vi "RichToFlatcif_manager_PluginInfoArray.vi"(5 "OutputClusterType":T1, 11 "InputCluster":T15) -> (3 "OutputCluster":T1)   [LabVIEW 2021, in "CIF_Manager_server.lvlib"]
uses:
  CIF_Manager_server.lvlib
  cif_manager_PluginInfoArray.ctl
  cif_manager_PluginInfo.ctl
  cif_common_ShortVersion.ctl
  cif_management_common_PluginStatusData.ctl
  cif_management_common_PluginStatusData_PluginState.ctl
  cif_management_common_TimingStatistics.ctl
  cif_common_TimingStats.ctl
  cif_management_common_FifoStatistics.ctl
  cif_management_common_Error.ctl
  cif_management_common_MonitorDoubles.ctl
  cif_management_common_MonitorU64.ctl
  cif_management_common_MonitorI64.ctl
  cif_management_common_LoaderInfo.ctl
  cif_management_common_LoaderType.ctl
  cif_manager_PluginInfoArray_Flat.ctl
  cif_manager_PluginInfo_Flat.ctl
  cif_common_ShortVersion_Flat.ctl
  cif_management_common_PluginStatusData_Flat.ctl
  cif_management_common_TimingStatistics_Flat.ctl
  cif_common_TimingStats_Flat.ctl
  cif_management_common_FifoStatistics_Flat.ctl
  cif_management_common_Error_Flat.ctl
  cif_management_common_MonitorDoubles_Flat.ctl
  cif_management_common_MonitorU64_Flat.ctl
  cif_management_common_MonitorI64_Flat.ctl
  cif_management_common_LoaderInfo_Flat.ctl
  RichToFlatcif_common_ShortVersion.vi
  RichToFlatcif_management_common_PluginStatusData.vi
  RichToFlatcif_management_common_LoaderInfo.vi
  RichToFlatcif_management_common_TimingStatistics.vi
  RichToFlatcif_management_common_FifoStatistics.vi
  RichToFlatcif_management_common_Error.vi
  RichToFlatcif_management_common_MonitorDoubles.vi
  RichToFlatcif_management_common_MonitorU64.vi
  RichToFlatcif_management_common_MonitorI64.vi
  RichToFlatcif_common_TimingStats.vi
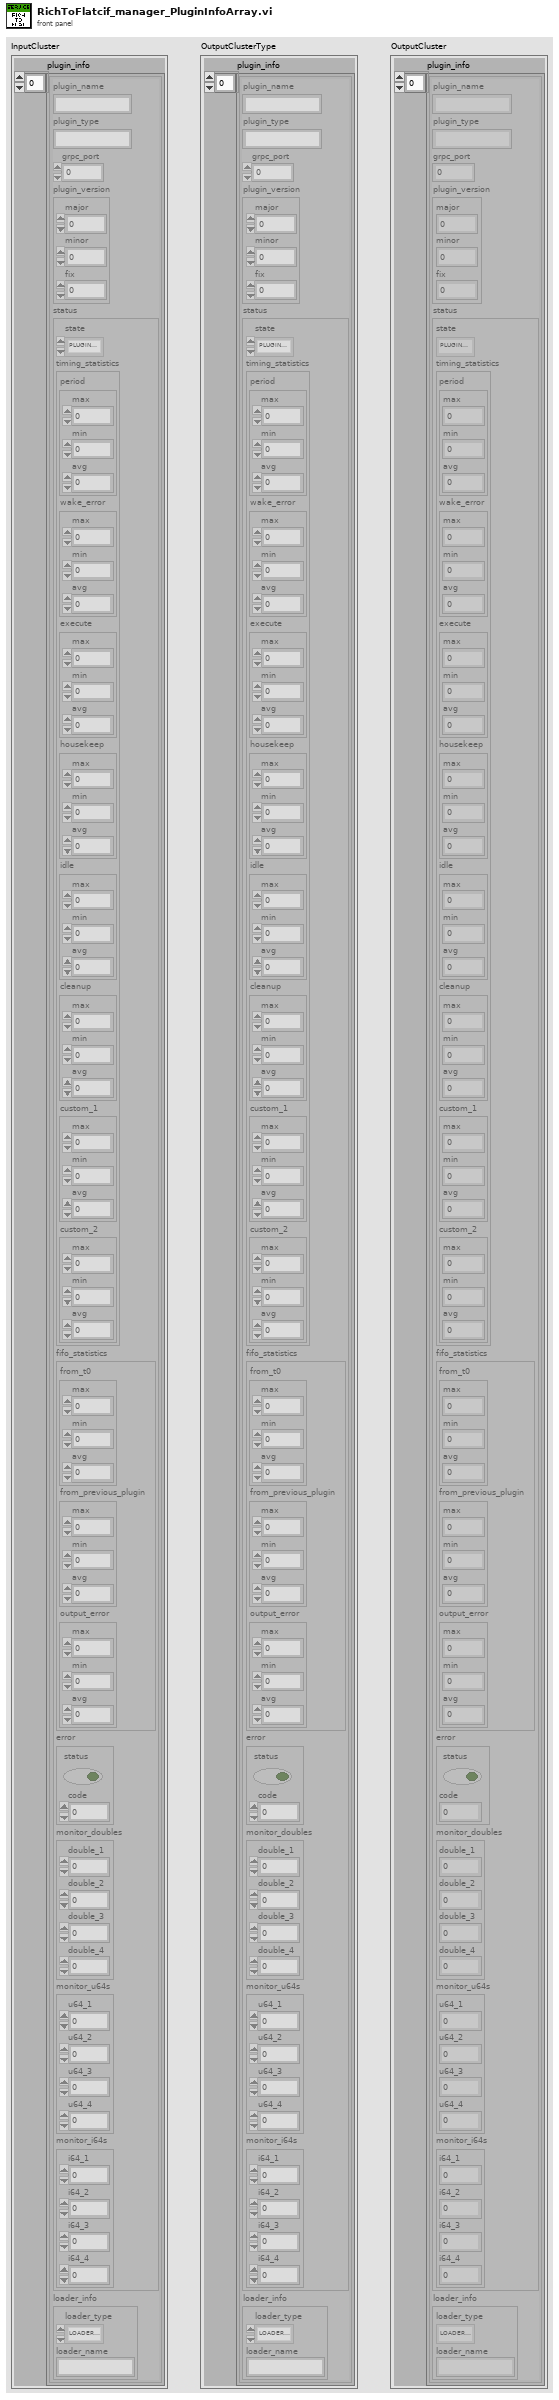
[diagram p1: front panel]
types:
  T1 = typedef "CIF_Manager_server.lvlib/cif_manager_PluginInfoArray_Flat.ctl" = cluster{"plugin_info":T2[]}
  T2 = typedef "CIF_Manager_server.lvlib/cif_manager_PluginInfo_Flat.ctl" = cluster{"plugin_name":string, "plugin_type":string, "grpc_port":i32, "plugin_version":T3, "status":T4, "loader_info":T13}
  T3 = typedef "CIF_Manager_server.lvlib/cif_common_ShortVersion_Flat.ctl" = cluster{"major":u32, "minor":u32, "fix":u32}
  T4 = typedef "CIF_Manager_server.lvlib/cif_management_common_PluginStatusData_Flat.ctl" = cluster{"state":T5, "timing_statistics":T6, "fifo_statistics":T8, "error":T9, "monitor_doubles":T10, "monitor_u64s":T11, "monitor_i64s":T12}
  T5 = typedef "CIF_Manager_server.lvlib/cif_management_common_PluginStatusData_PluginState.ctl" = enum32{"PLUGINSTATE_UNKNOWN", "PLUGINSTATE_CREATING", "PLUGINSTATE_LISTENING", "PLUGINSTATE_RUNNING", "PLUGINSTATE_CLEANINGUP", "PLUGINSTATE_DESTROYING", "PLUGINSTATE_PREPARED", "PLUGINSTATE_FTE_RUN"}
  T6 = typedef "CIF_Manager_server.lvlib/cif_management_common_TimingStatistics_Flat.ctl" = cluster{"period":T7, "wake_error":T7, "execute":T7, "housekeep":T7, "idle":T7, "cleanup":T7, "custom_1":T7, "custom_2":T7}
  T7 = typedef "CIF_Manager_server.lvlib/cif_common_TimingStats_Flat.ctl" = cluster{"max":i64, "min":i64, "avg":dbl}
  T8 = typedef "CIF_Manager_server.lvlib/cif_management_common_FifoStatistics_Flat.ctl" = cluster{"from_t0":T7, "from_previous_plugin":T7, "output_error":T7}
  T9 = typedef "CIF_Manager_server.lvlib/cif_management_common_Error_Flat.ctl" = cluster{"status":bool, "code":i32}
  T10 = typedef "CIF_Manager_server.lvlib/cif_management_common_MonitorDoubles_Flat.ctl" = cluster{"double_1":dbl, "double_2":dbl, "double_3":dbl, "double_4":dbl}
  T11 = typedef "CIF_Manager_server.lvlib/cif_management_common_MonitorU64_Flat.ctl" = cluster{"u64_1":u64, "u64_2":u64, "u64_3":u64, "u64_4":u64}
  T12 = typedef "CIF_Manager_server.lvlib/cif_management_common_MonitorI64_Flat.ctl" = cluster{"i64_1":i64, "i64_2":i64, "i64_3":i64, "i64_4":i64}
  T13 = typedef "CIF_Manager_server.lvlib/cif_management_common_LoaderInfo_Flat.ctl" = cluster{"loader_type":T14, "loader_name":string}
  T14 = typedef "CIF_Manager_server.lvlib/cif_management_common_LoaderType.ctl" = enum32{"LOADERTYPE_UNKNOWN", "LOADERTYPE_LABVIEW"}
  T15 = typedef "CIF_Manager_server.lvlib/cif_manager_PluginInfoArray.ctl" = cluster{"plugin_info":T16[]}
  T16 = typedef "CIF_Manager_server.lvlib/cif_manager_PluginInfo.ctl" = cluster{"plugin_name":string, "plugin_type":string, "grpc_port":i32, "plugin_version":T17, "status":T18, "loader_info":T26}
  T17 = typedef "CIF_Manager_server.lvlib/cif_common_ShortVersion.ctl" = cluster{"major":u32, "minor":u32, "fix":u32}
  T18 = typedef "CIF_Manager_server.lvlib/cif_management_common_PluginStatusData.ctl" = cluster{"state":T5, "timing_statistics":T19, "fifo_statistics":T21, "error":T22, "monitor_doubles":T23, "monitor_u64s":T24, "monitor_i64s":T25}
  T19 = typedef "CIF_Manager_server.lvlib/cif_management_common_TimingStatistics.ctl" = cluster{"period":T20, "wake_error":T20, "execute":T20, "housekeep":T20, "idle":T20, "cleanup":T20, "custom_1":T20, "custom_2":T20}
  T20 = typedef "CIF_Manager_server.lvlib/cif_common_TimingStats.ctl" = cluster{"max":i64, "min":i64, "avg":dbl}
  T21 = typedef "CIF_Manager_server.lvlib/cif_management_common_FifoStatistics.ctl" = cluster{"from_t0":T20, "from_previous_plugin":T20, "output_error":T20}
  T22 = typedef "CIF_Manager_server.lvlib/cif_management_common_Error.ctl" = cluster{"status":bool, "code":i32}
  T23 = typedef "CIF_Manager_server.lvlib/cif_management_common_MonitorDoubles.ctl" = cluster{"double_1":dbl, "double_2":dbl, "double_3":dbl, "double_4":dbl}
  T24 = typedef "CIF_Manager_server.lvlib/cif_management_common_MonitorU64.ctl" = cluster{"u64_1":u64, "u64_2":u64, "u64_3":u64, "u64_4":u64}
  T25 = typedef "CIF_Manager_server.lvlib/cif_management_common_MonitorI64.ctl" = cluster{"i64_1":i64, "i64_2":i64, "i64_3":i64, "i64_4":i64}
  T26 = typedef "CIF_Manager_server.lvlib/cif_management_common_LoaderInfo.ctl" = cluster{"loader_type":T14, "loader_name":string}
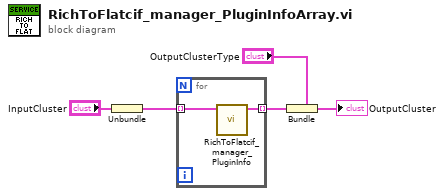
[diagram p0: block diagram]
diagram:
  n1 = Unbundle "Unbundle"("InputCluster") -> ("plugin_info"=w2:T16[])
  n2 = for {
    tunnel: w2 -> [w7] mode=indexing
    tunnel: [w6] -> w1 mode=indexing
    n3 = call "RichToFlatcif_manager_PluginInfo.vi"("InputCluster"=w7) -> ("OutputCluster"=w6:T2)  [unwired: 10 in]
  }
  n4 = Bundle "Bundle"(cluster="OutputClusterType", "plugin_info"=w1) -> (→"OutputCluster":T1)
